vi "Test Latest Received Message is Returned.vi"(8 "error in (no error)":errorcluster, 11 "Test Case In":refnum<class "Debug Latest Message Test.lvclass">) -> (0 "error out":errorcluster, 3 "Test Case Out":refnum<class "Debug Latest Message Test.lvclass">)   [LabVIEW 2020, in "Debug Latest Message Test.lvclass"]
uses:
  Debug Latest Message Test.lvclass
  C:/Program Files (x86)/National Instruments/LabVIEW 2020/vi.lib/Astemes/LUnit/Test Case.lvclass
  source/Debug Latest Message/Debug Latest Message.lvclass
  source/Debug Data/Raw Debug Data.ctl
  <vilib>/Astemes/LUnit/Test Case.lvclass/Test Case.ctl
  <vilib>/Astemes/LUnit/LUnit Assertion Result.lvclass/LUnit Assertion Result.ctl
  <vilib>/Astemes/LUnit/LUnit Test Case Result.lvclass/LUnit Test Case Result.ctl
  <vilib>/Astemes/LUnit/LUnit Method Result.lvclass/LUnit Method Result.ctl
  01074fa8-ee8a-411d-bc8b-fc92c4f90959.vi
  <vilib>/Astemes/LUnit/Palette/Pass.vi
  <vilib>/Astemes/LUnit/Palette/Fail.vi
  <vilib>/Astemes/LUnit/Compare Variants.vi
  <vilib>/Astemes/LUnit/Describe Comparison.vi
  <vilib>/Astemes/LUnit/Set Assertion Type.vi
  <vilib>/Astemes/LUnit/Add test result.vi
  <vilib>/Astemes/LUnit/LUnit Write Passed.vi
  <vilib>/Astemes/LUnit/LUnit Write Message.vi
  <vilib>/Astemes/LUnit/LUnit Write Description.vi
  <vilib>/Astemes/LUnit/Variant to string.vi
  <vilib>/Astemes/LUnit/LUnit Write Assertion Type.vi
  <vilib>/Astemes/LUnit/LUnit Record Assertion Result.vi
  <vilib>/Astemes/LUnit/LUnit Aggregate Assertion Results.vi
  <vilib>/Astemes/LUnit/Assertion Result/LUnit Read Status.vi
  <vilib>/Astemes/LUnit/LUnit Read Message.vi
  <vilib>/Astemes/LUnit/LUnit Read Description.vi
  <vilib>/Astemes/LUnit/Method Result/LUnit Merge Status.vi
  <vilib>/Astemes/LUnit/LUnit Concatenate result strings.vi
  <vilib>/Utility/Data Type/Get Type Information.vi
  <vilib>/Utility/LVClass/Get LV Class Name.vi
  <vilib>/Astemes/LUnit/LUnit Assertion Result.lvclass
  source/Debug Data/Debug Data.lvclass
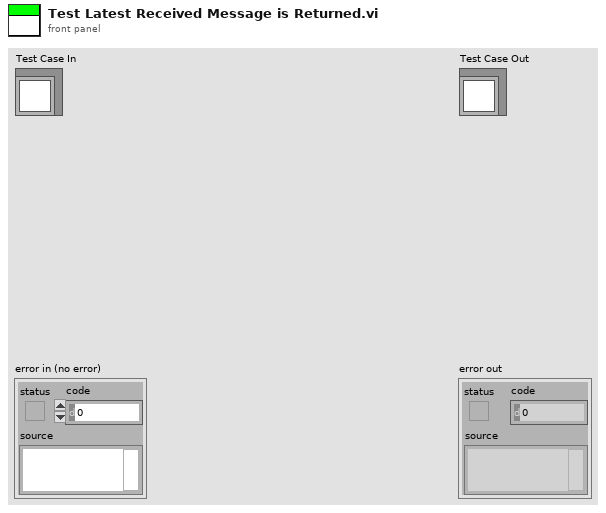
[diagram p1: front panel]
types:
  T1 = typedef "Debug Data.lvclass/Raw Debug Data.ctl" = cluster{"Action":string, "Call Chain":string, "Process":string, "Message":string, "Message Data":variant, "Time":dbl}
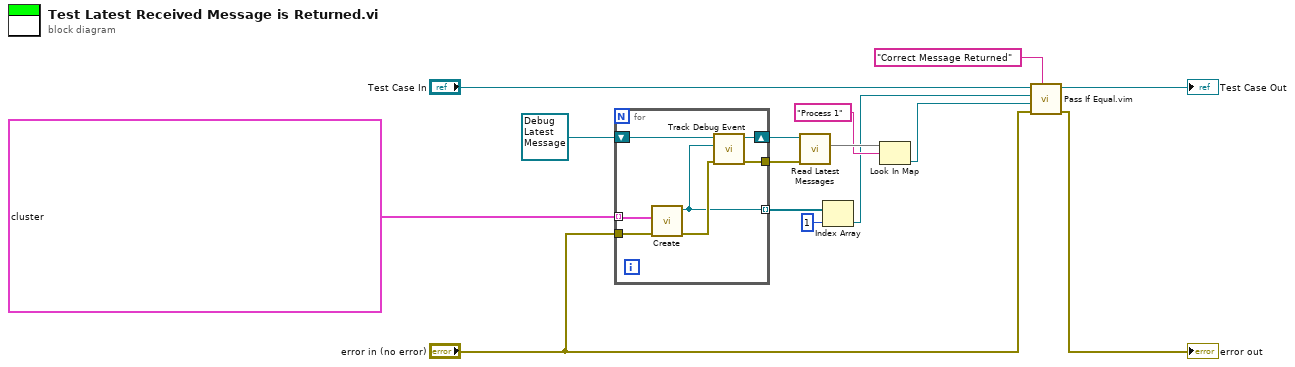
[diagram p0: block diagram]
diagram:
  n1 = for {
    tunnel: [w21] -> w11
    shift-right: [w22] -> w12
    shift-left: refnum<class "Debug Latest Message.lvclass"> refnum ("Debug Latest Message in") -> [w20]
    tunnel: T1[] [{"Action"="Send", "Call Chain"="Test.vi:123456", "Process"="Process 1", "Message"="Init", "Message Data"=variant, "Time"=0.0}, {"Action"="Receive", "Call Chain"="TF.lvlib:Process.lvclass:Handle Messages.vi:1960001", "Process"="Process 1", "Message"="Init", "Message Data"=variant, "Time"=0.0}, {"Action"="Send", "Call Chain"="Test.vi", "Process"="Process 1", "Message"="Start", "Message Data"=variant, "Time"=0.0}] ("Debug Data Cluster") -> [w19] mode=indexing
    tunnel: "error in (no error)" -> [w18]
    tunnel: [w16] -> w7 mode=indexing
    n2 = call "Create.vi"("error in (no error)"=w18, "Debug Data Cluster"=w19) -> ("error out"=w17:errorcluster, "Debug Data out"=w16:refnum<class "Debug Data.lvclass">)  [unwired: 8 in]
    n3 = call "Track Debug Event.vi"("error in (no error)"=w17, "Debug Data.lvclass"=w16, "Debug Latest Message In"=w20) -> ("error out"=w21:errorcluster, "Debug Latest Message Out"=w22:refnum<class "Debug Latest Message.lvclass">)  [unwired: 7 in]
  }
  n4 = call "Read Latest Messages.vi"("error in (no error)"=w11, "Debug Latest Message in"=w12) -> ("Latest Messages"=w6:map{string, refnum<class "Debug Data.lvclass">})  [unwired: 7 in, 2 out]
  n5 = Index Array(array=w7, index=1) -> (element=w2:refnum<class "Debug Data.lvclass">)
  n6 = Look In Map(map=w6, key="Process 1") -> (value=w3:refnum<class "Debug Data.lvclass">)  [unwired: 1 in, 1 out]
  n7 = call "Pass If Equal.vim"("Description"="Correct Message Returned", "error in (no error)"="error in (no error)", "Actual"=w3, "Expected"=w2, "LUnit Test Case In"="Test Case In") -> ("error out"=→"error out":errorcluster, "LUnit Test Case Out"=→"Test Case Out":refnum<class "Debug Latest Message Test.lvclass">)  [unwired: 5 in]
